vi "in_range_plus_minus.vi"(8 "error in (no error)":errorcluster, 9 "in":dbl, 10 "+/-":dbl, 11 "x":dbl) -> (0 "error out":errorcluster, 3 "in_range":bool)   [LabVIEW 2020]
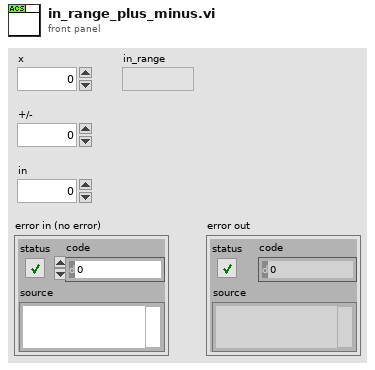
[diagram p1: front panel]
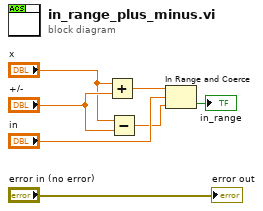
[diagram p0: block diagram]
diagram:
  n1 = Add(x="x", y="+/-") -> (x+y=w4:dbl)
  n2 = Subtract(x="x", y="+/-") -> (x-y=w5:dbl)
  n3 = In Range and Coerce(upper limit=w4, x="in", lower limit=w5) -> (In Range?=→"in_range":bool)  [unwired: 1 out]
  "error out" <- "error in (no error)"
